vi "Initialize.vi"(0 "Display State In":T2, 5 "Channel Names":string[](array[string]), 7 "Previous Channels Names":string[](array[string]), 9 "Container State":T3, 11 "error in (no error)":errorcluster, 12 "Data Valid":T1) -> (4 "Display State Out":T2, 15 "error out":errorcluster)   [LabVIEW 2021, in "myRIO Channel Name.xctl"]
uses:
  <vilib>/myRIO/Common/Express VI Framework/xctls/myRIO Channel Name/myRIO Channel Name.xctl
  <vilib>/_xctls/Container State.ctl
  <vilib>/myRIO/Common/Express VI Framework/xctls/myRIO Channel Name/State.ctl
  <vilib>/myRIO/Common/Express VI Framework/typedefs/Data Validate Ref.ctl
  <vilib>/_xctls/XControlSupport.lvlib
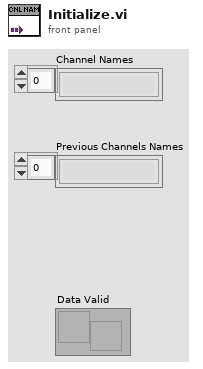
[diagram p1: front panel]
types:
  T1 = typedef "Data Validate Ref.ctl" = refnum<user-event>
  T2 = typedef "myRIO Channel Name.xctl/State.ctl" = cluster{"Channel Names":string[], "Data Valid":T1, "Current Channel":string}
  T3 = typedef "XControlSupport.lvlib/Container State.ctl" = cluster{"Indicator?":bool, "Run Mode?":bool, " Refnum":refnum<vi>}
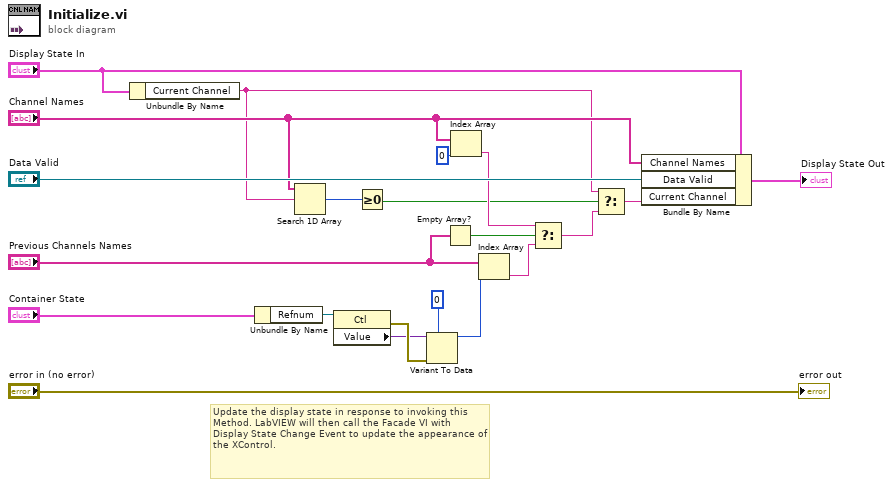
[diagram p0: block diagram]
diagram:
  # "Update the display state in response to invoking this Method. LabVIEW will then call the Facade VI with Display State Change Event to update the appearance of the XControl."
  n1 = Unbundle By Name("Display State In") -> ("Current Channel"=w5:string)
  n2 = Unbundle By Name("Container State") -> ("Refnum"=w17:refnum<vi>)
  n3 = Search 1D Array(1D array="Channel Names", element=w5) -> (index of element=w7:i32)  [unwired: 1 in]
  n4 = property class="Ctl"(reference=w17) -> (error out=w15:errorcluster, "Value"=w14:variant)  [unwired: 1 in, 1 out]
  n5 = Greater Or Equal To 0?(x=w7) -> (x >= 0?=w6:bool)
  n6 = Variant To Data(error in=w15, type=u32 0, Variant=w14) -> (data=w1:u32)  [unwired: 1 out]
  n7 = Empty Array?(array="Previous Channels Names") -> (empty?=w13:bool)
  n8 = Index Array(array="Channel Names", index=0) -> (element=w11:string)
  n9 = Index Array(array="Previous Channels Names", index=w1) -> (element=w9:string)
  n10 = Select(t=w11, s=w13, f=w9) -> (s? t:f=w4:string)
  n11 = Select(t=w5, s=w6, f=w4) -> (s? t:f=w3:string)
  n12 = Bundle By Name(cluster="Display State In", "Channel Names"="Channel Names", "Data Valid"="Data Valid", "Current Channel"=w3) -> (→"Display State Out":T2)
  "error out" <- "error in (no error)"
